vi "FrontPanel_Control.vi"(8 "error in (no error)":errorcluster, 10 "FP_open?":bool=TRUE, 11 "MonSys_Server_Actor in":refnum<class "MonSys_Server_Actor.lvclass">) -> (0 "error out":errorcluster, 3 "MonSys_Server_Actor out":refnum<class "MonSys_Server_Actor.lvclass">)   [LabVIEW 2018, in "MonSys_Server_Actor.lvlib" / "MonSys_Server_Actor.lvclass"]
doc: "fire FP contorl event -> to open or close FP"
uses:
  MonSys_Server_Actor.lvclass
  MonSys_Server_Actor.lvclass/MonSys_Server_Actor.ctl
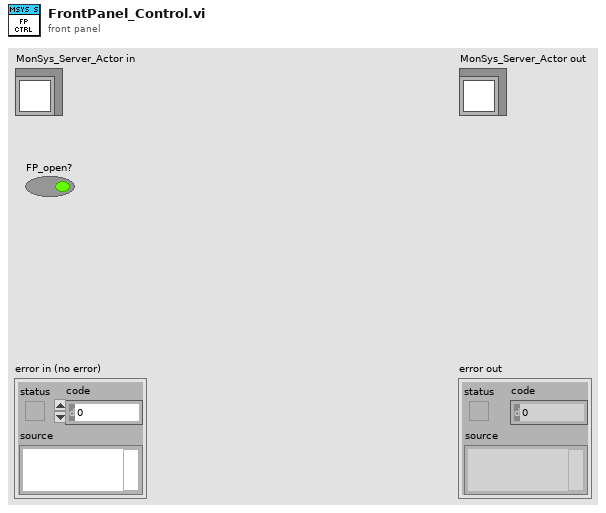
[diagram p1: front panel]
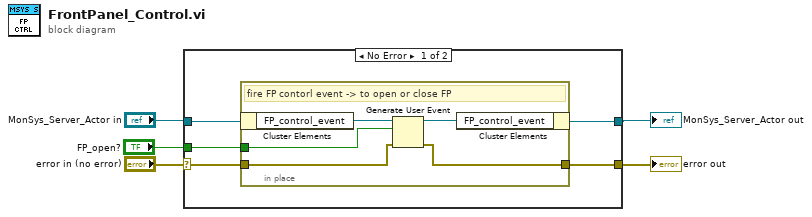
[diagram p0: block diagram]
diagram:
  n1 = case shown="No Error" "error in (no error)" {
    selector: "error in (no error)" -> [w6 w17]
    tunnel: [w9 w17] -> w3
    tunnel: [w8 w16] -> w2
    tunnel: "MonSys_Server_Actor in" -> [w10 w16]
    tunnel: "FP_open?" -> [w7 _]
    frame No Error {
      n2 = in-place {
        in-place-border: [w11] -> w9
        in-place-border: w7 -> [w15]
        in-place-border: w6 -> [w12]
        # "fire FP contorl event -> to open or close FP"
        n3 = in-place-cluster #1(w10) -> ("FP_control_event"=w14:refnum<user-event>)
        n4 = Generate User Event(user event=w14, event data cluster=w15, error in=w12) -> (user event out=w13:refnum<user-event>, error out=w11:errorcluster)  [unwired: 1 in]
        n5 = in-place-cluster #1("FP_control_event"=w13) -> (w8:refnum<class "MonSys_Server_Actor.lvclass">)
      }
    }
    frame Error {
    }
  }
  "error out" <- w3
  "MonSys_Server_Actor out" <- w2
